vi "FPposition.vi"(3 "VI Ref":refnum<vi>, 4 "Action":enum16{"Make string", "Decode string"}(ring), 5 "String In":string) -> (0 "left":i32, 1 "top":i32, 2 "String Out":string)   [LabVIEW 2014]
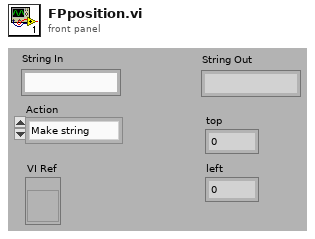
[diagram p1: front panel]
types:
  T1 = typedef "LVRectTypeDef.ctl" = cluster{"Left":i16, "Top":i16, "Right":i16, "Bottom":i16}
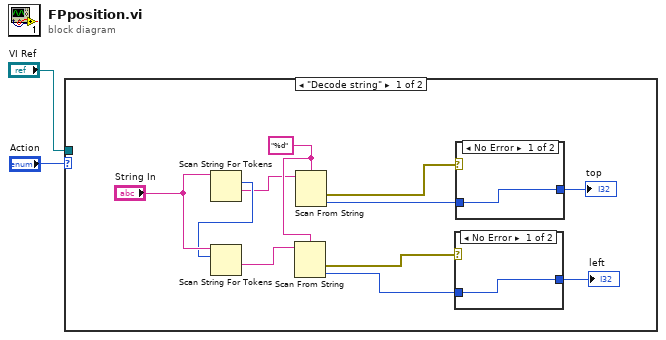
[diagram p0: block diagram]
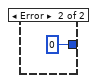
[diagram p2: hidden frame]
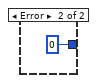
[diagram p3: hidden frame]
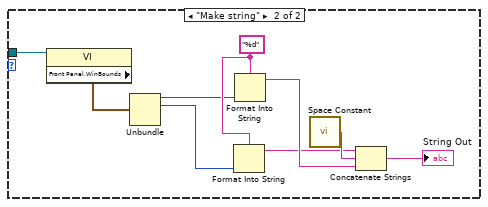
[diagram p4: hidden frame]
diagram:
  n1 = case shown="\"Decode string\"" "Action" {
    tunnel: "VI Ref" -> [_ w18]
    frame "Decode string" {
      w11 = "%d" ("format string")
      n2 = Scan String For Tokens(9:"String In") -> (1:w10:string, 2:w12:i32)  [unwired: 5 in, 2 out]
      n3 = Scan String For Tokens(8:w12, 9:"String In") -> (1:w9:string)  [unwired: 4 in, 3 out]
      n4 = Scan From String(format string=w11, input string=w9) -> (error out=w3:errorcluster, output 1=w4:i32)  [unwired: 3 in, 2 out]
      n5 = Scan From String(format string=w11, input string=w10) -> (error out=w8:errorcluster, output 1=w6:i32)  [unwired: 3 in, 2 out]
      n6 = case shown="No Error" w3 {
        tunnel: [w14 0] -> w5
        tunnel: w4 -> [w14 _]
        frame No Error {
        }
        frame Error {
        }
      }
      "left" <- w5
      n7 = case shown="No Error" w8 {
        tunnel: [w16 0] -> w7
        tunnel: w6 -> [w16 _]
        frame No Error {
        }
        frame Error {
        }
      }
      "top" <- w7
    }
    frame "Make string" {
      w26 = "%d" ("format string")
      n8 = property class="VI"(reference=w18) -> ("Front Panel.WinBounds"=w19:T1)  [unwired: 1 in, 2 out]
      n9 = Unbundle(w19) -> ("Left"=w25:i16, "Top"=w24:i16)  [unwired: 2 out]
      n10 = Format Into String(format string=w26, w24) -> (resulting string=w20:string)  [unwired: 2 in, 1 out]
      n11 = Format Into String(format string=w26, w25) -> (resulting string=w21:string)  [unwired: 2 in, 1 out]
      n12 = call <vilib>:"Space Constant.vi"() -> ("String"=w22:string)
      n13 = Concatenate Strings(w20, w22, w21) -> (→"String Out":string)
    }
  }
